vi "SignalGenerator.vi"(9 "Stop":bool, 10 "Signal Parameters":cluster{"Frequency":dbl, "Amplitude":dbl}) -> ()   [LabVIEW 2014]
panel:
  out "error out":errorcluster
  out "error in":errorcluster
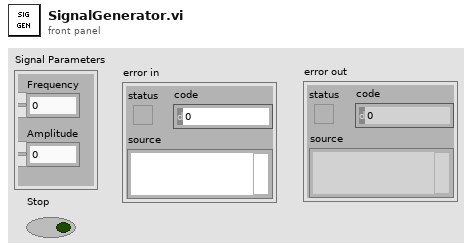
[diagram p1: front panel]
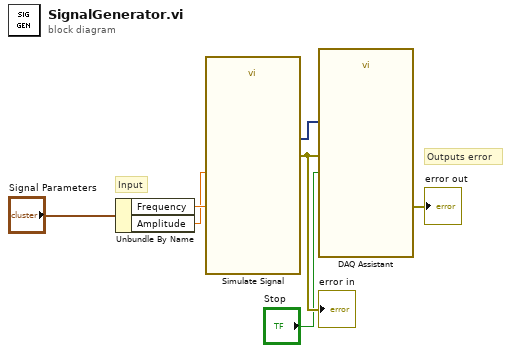
[diagram p0: block diagram]
diagram:
  # "Outputs error"
  # "Input"
  n1 = Unbundle By Name("Signal Parameters") -> ("Frequency"=w2:dbl, "Amplitude"=w1:dbl)
  n2 = call "Simulate Signal"("Frequency"=w2, "Amplitude"=w1) -> ("Sine"=w5:dynamicdata, "error out"=w7:errorcluster)  [unwired: 12 in]
  "error in" <- w7
  n3 = call "DAQ Assistant"("data"=w5, "error in"=w7, "stop (F)"="Stop") -> ("error out"=→"error out":errorcluster)  [unwired: 14 in, 2 out]
